vi "NI VeriStand - Add Custom Device Section.vi"(4 "Property Values":variant[](array[variant]), 5 "Highlight? (F)":bool, 6 "Property names":string[](array[string]), 7 "GUID (Default Section)":string="03D3BB89-1485-13A6-56005DE6430FF8B7", 8 "error in (no error)":errorcluster, 10 "Section Name":string, 11 "Parent Ref in":T1 format="%.0x") -> (0 "error out":errorcluster, 1 "Section Ptr":T1 format="%.0x", 2 "Newly Created?":bool, 3 "Parent Ref out":T1 format="%.0x")   [LabVIEW 2020, in "Custom Device API.lvlib"]
doc: "Adds a section with the name <B>Section Name</B> to the device specified by <B>Parent Ref in</B>. If the <B>Section Name</B> you specify already exists for that device, this VI updates the page <B>GUID</B> and the values of any properties."
uses:
  <vilib>/NI VeriStand/Custom Device API/Custom Device API.lvlib
  <vilib>/NI VeriStand/Custom Device API/Custom Device Item Ref.ctl
  e6ab5371-927d-4749-b9b0-4dfc5222fed8.vi
  <vilib>/NI VeriStand/Custom Device API/Custom Device Offline Path.vi
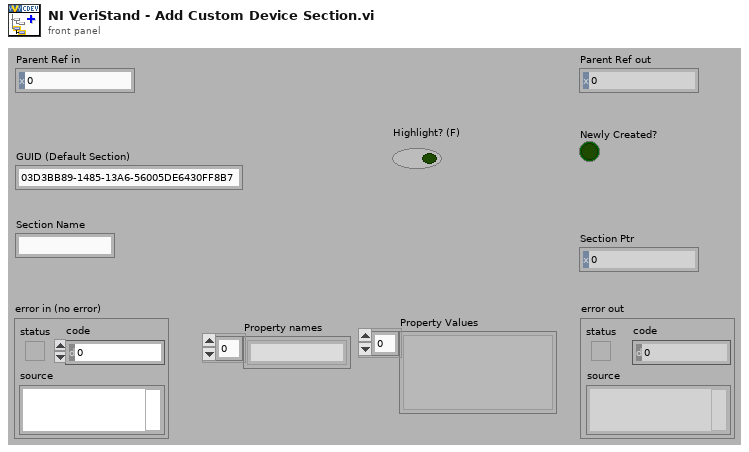
[diagram p1: front panel]
types:
  T1 = typedef "Custom Device API.lvlib/Custom Device Item Ref.ctl" = u64
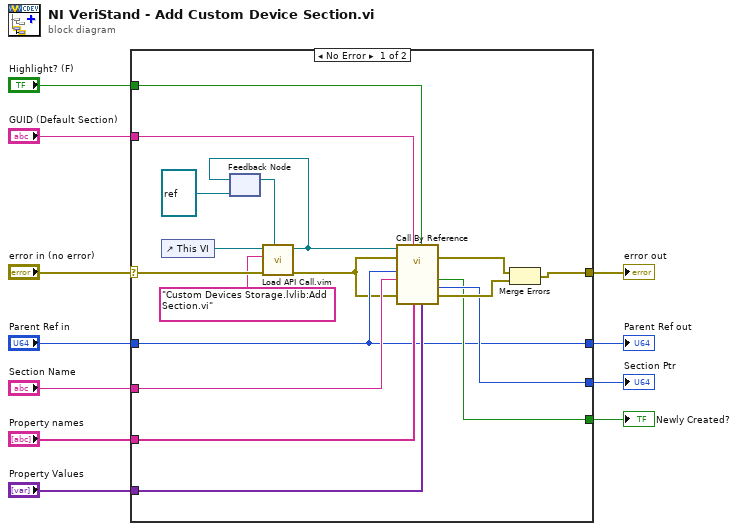
[diagram p0: block diagram]
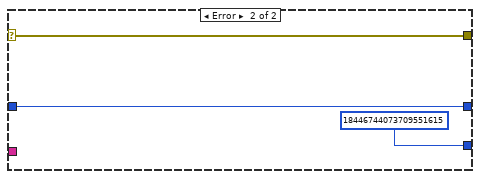
[diagram p2: hidden frame]
diagram:
  n1 = case shown="No Error" "error in (no error)" {
    selector: "error in (no error)" -> [w17 w31]
    tunnel: [w28 w31] -> w11
    tunnel: [w27 T1 18446744073709551615 ("Channel Ref")] -> w10
    tunnel: [w20 w32] -> w9
    tunnel: "Highlight? (F)" -> [w26 _]
    tunnel: "GUID (Default Section)" -> [w25 _]
    tunnel: "Parent Ref in" -> [w20 w32]
    tunnel: "Section Name" -> [w24 _]
    tunnel: "Property names" -> [w23 _]
    tunnel: "Property Values" -> [w22 _]
    tunnel: [w21 _] -> w2
    frame No Error {
      n2 = control-ref of="This VI"() -> (w18:refnum<vi>)
      n3 = feedback #1(refnum<vi> refnum ("type specifier VI Refnum (for type only)")) -> (w19:refnum<vi>)
      n4 = call "Load API Call.vim"("VI reference in"=w19, "error in (no error)"=w17, "VI qualified name"="Custom Devices Storage.lvlib:Add Section.vi", "Caller VI ref"=w18) -> ("error out"=w16:errorcluster, "VI reference"=w15:refnum<vi>)  [unwired: 6 in]
      n5 = feedback-in #1(w15) -> ()
      n6 = call-by-ref "?"(reference=w15, error in=w16, "Property Values"=w22, "Highlight? (F)"=w26, "Property names"=w23, "GUID (Default Section)"=w25, 8:"error in (no error)"=w16, "Section Name"=w24, "Parent Ref in"=w20) -> (error out=w12:errorcluster, 0:"error out"=w29:errorcluster, "Section Ptr"=w27:T1, "Newly Created?"=w21:bool)  [unwired: 1 in, 2 out]
      n7 = Merge Errors(w12, w29) -> (w28:errorcluster)
    }
    frame Error {
    }
  }
  "error out" <- w11
  "Parent Ref out" <- w9
  "Section Ptr" <- w10
  "Newly Created?" <- w2
